vi "RSZVB Set Sweep Segment Spur Avoid.vi"(7 "Spur Avoid (Positive)":i32(ring) items=["Positive", "Negative", "Auto"], 8 "error in (no error)":errorcluster {"code" format="%.0x"}, 9 "Segment (1)":i32=1, 10 "Channel (1)":i32=1, 11 "VISA session":refnum<visa-resource-name>) -> (0 "error out":errorcluster {"code" format="%.0x"}, 3 "dup VISA session":refnum<visa-resource-name>)   [LabVIEW 2011]
doc: "This VI defines the position of the local oscillator frequency LO relative to the RF frequency (sideband, Spur Avoid) in sweep segment no. <Seg>. \n\nRemote-control command(s):\n[SENSe<Ch>:]SEGMent<Seg>:SBANd"
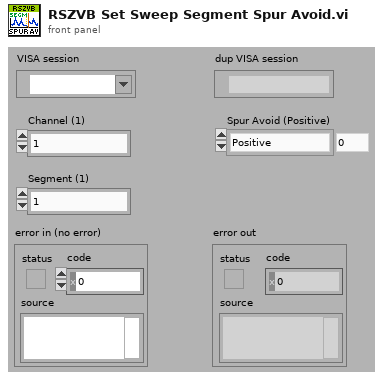
[diagram p1: front panel]
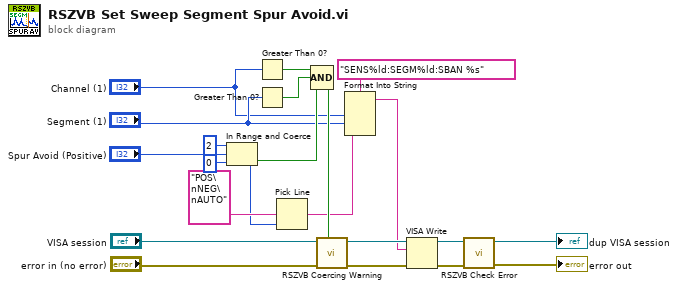
[diagram p0: block diagram]
diagram:
  n1 = In Range and Coerce(upper limit=2, x="Spur Avoid (Positive)", lower limit=0) -> (coerced(x)=w9:i32, In Range?=w11:bool)
  n2 = Greater Than 0?(x="Channel (1)") -> (x > 0?=w15:bool)
  n3 = Greater Than 0?(x="Segment (1)") -> (x > 0?=w14:bool)
  n4 = Pick Line(multi-line string="POS\nNEG\nAUTO", line index=w9) -> (output string=w8:string)  [unwired: 1 in]
  n5 = Compound Arithmetic op=AND(w15, w14, w11) -> (w17:bool)
  n6 = call "RSZVB Coercing Warning.vi"("In Range?"=w17, "error in (no error)"="error in (no error)", "VISA session"="VISA session") -> ("error out"=w20:errorcluster, "dup VISA session"=w21:refnum<visa-resource-name>)  [unwired: 7 in]
  n7 = Format Into String(format string="SENS%ld:SEGM%ld:SBAN %s", "Channel (1)", "Segment (1)", w8) -> (resulting string=w16:string)  [unwired: 2 in, 1 out]
  n8 = VISA Write(VISA resource name=w21, write buffer=w16, error in (no error)=w20) -> (VISA resource name out=w18:refnum<visa-resource-name>, error out=w19:errorcluster)  [unwired: 1 out]
  n9 = call "RSZVB Check Error.vi"("error in (no error)"=w19, "VISA session"=w18) -> ("error out"=→"error out":errorcluster, "dup VISA session"=→"dup VISA session":refnum<visa-resource-name>)  [unwired: 8 in]
